vi "Proyectocalculadora.vi"() -> ()   [LabVIEW 2020]
panel:
  in  "?":bool
  out "RESULTADOS":dbl
  in  "VALOR Y":dbl
  in  "VALOR  X":dbl
  in  "OPERACIONES":T1(ring)
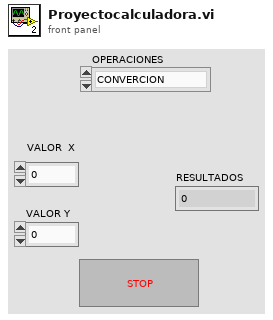
[diagram p1: front panel]
types:
  T1 = enum16{"CONVERCION", "TANGENTE", "COSENO", "SENO", "EXPONENCIAL", "RAIZ", "DIVICION", "MULTIPLICACION", "RESTA", "SUMA"}
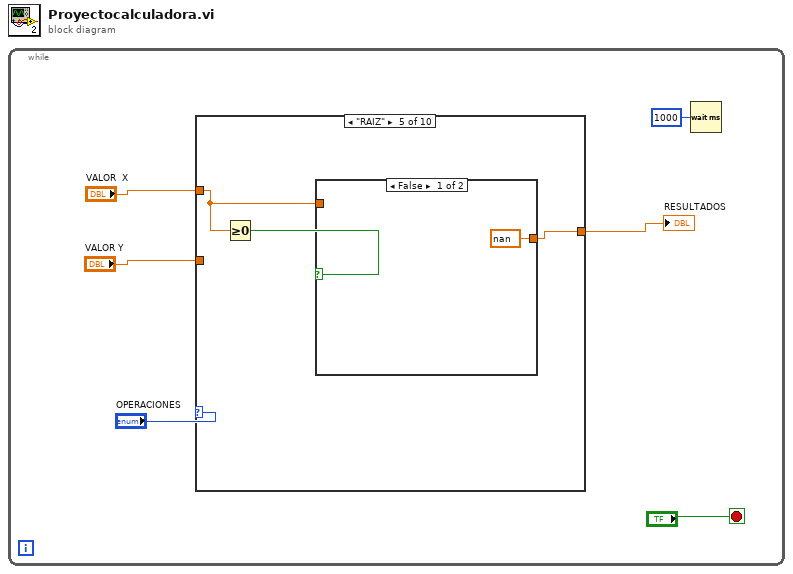
[diagram p0: block diagram]
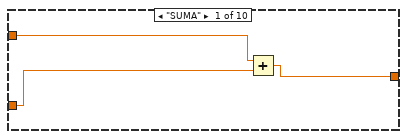
[diagram p2: hidden frame]
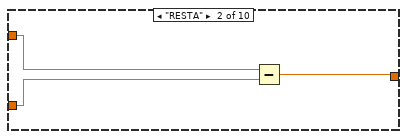
[diagram p3: hidden frame]
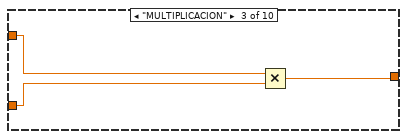
[diagram p4: hidden frame]
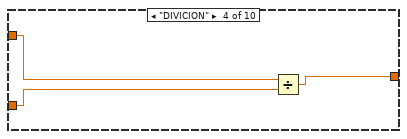
[diagram p5: hidden frame]
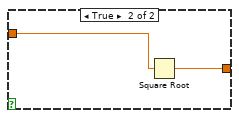
[diagram p6: hidden frame]
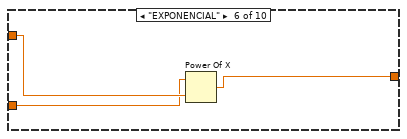
[diagram p7: hidden frame]
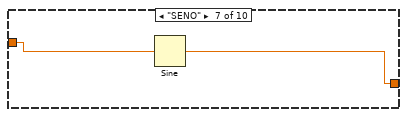
[diagram p8: hidden frame]
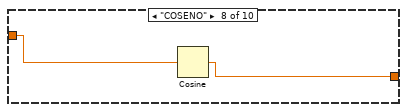
[diagram p9: hidden frame]
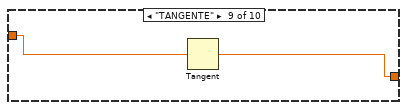
[diagram p10: hidden frame]
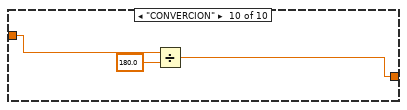
[diagram p11: hidden frame]
diagram:
  n1 = while {
    stop <- "?" stop-if-true
    n2 = case shown="\"RAIZ\"" "OPERACIONES" {
      tunnel: "VALOR  X" -> [w8 w12 w15 w18 w20 w27 w28 w31 w33 w36]
      tunnel: "VALOR Y" -> [w7 w11 w14 w17 _ w26 _ _ _ _]
      tunnel: [w9 w10 w13 w16 w19 w25 w29 w30 w32 w34] -> w4
      frame "SUMA" {
        n3 = Add(x=w8, y=w7) -> (x+y=w9:dbl)
      }
      frame "RESTA" {
        n4 = Subtract(x=w12, y=w11) -> (x-y=w10:dbl)
      }
      frame "MULTIPLICACION" {
        n5 = Multiply(x=w15, y=w14) -> (x*y=w13:dbl)
      }
      frame "DIVICION" {
        n6 = Divide(x=w18, y=w17) -> (x/y=w16:dbl)
      }
      frame "RAIZ" {
        n7 = Greater Or Equal To 0?(x=w20) -> (x >= 0?=w21:bool)
        n8 = case shown="False" w21 {
          tunnel: w20 -> [_ w24]
          tunnel: [nan w23] -> w19
          frame False {
          }
          frame True {
            n9 = Square Root(x=w24) -> (sqrt(x)=w23:dbl)
          }
        }
      }
      frame "EXPONENCIAL" {
        n10 = Power Of X(1:w27, 2:w26) -> (0:w25:dbl)
      }
      frame "SENO" {
        n11 = Sine(x=w28) -> (sin(x)=w29:dbl)
      }
      frame "COSENO" {
        n12 = Cosine(x=w31) -> (cos(x)=w30:dbl)
      }
      frame "TANGENTE" {
        n13 = Tangent(1:w33) -> (0:w32:dbl)
      }
      frame "CONVERCION" {
        n14 = Divide(x=w36, y=180.0) -> (x/y=w34:dbl)
      }
    }
    "RESULTADOS" <- w4
    n15 = Wait (ms)(milliseconds to wait=u32 1000) -> ()  [unwired: 1 out]
  }
